vi "scanalone count cards.vi"(8 "error in (no error)":errorcluster) -> (0 "error out":errorcluster, 3 "function return":u16)   [LabVIEW 2015, in "SCANalone4x64.lvlib"]
doc: "__declspec(dllimport) unsigned short __stdcall scanalone_count_cards(void);"
uses:
  <userlib>/SCANalone4x64/SCANalone4x64.lvlib
  <userlib>/SCANalone4x64/SCANalone4x64.dll
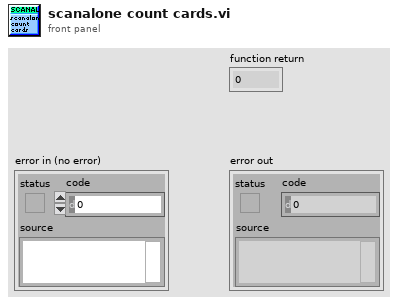
[diagram p1: front panel]
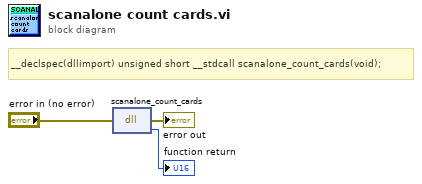
[diagram p0: block diagram]
diagram:
  # "__declspec(dllimport) unsigned short __stdcall scanalone_count_cards(void);"
  n1 = dll-call lib="C:/Program Files/National Instruments/LabVIEW 2015/user.lib/SCANalone4x64/SCANalone4x64.*" fn="scanalone_count_cards"(error in="error in (no error)") -> (error out=→"error out":errorcluster, →"function return":u16)  [unwired: 2 in, 1 out]
